vi "ReadWaveDataProcess.vi"(8 "error in (no error)":errorcluster, 11 "ScopeAA in":refnum<class "ScopeAA.lvclass">) -> (0 "error out":errorcluster, 2 "Waveform":waveform(dbl), 3 "ScopeAA out":refnum<class "ScopeAA.lvclass">)   [LabVIEW 2018, in "ScopeAA.lvclass"]
uses:
  ScopeAA.lvclass
  <vilib>/measure/NI_MABase.lvlib
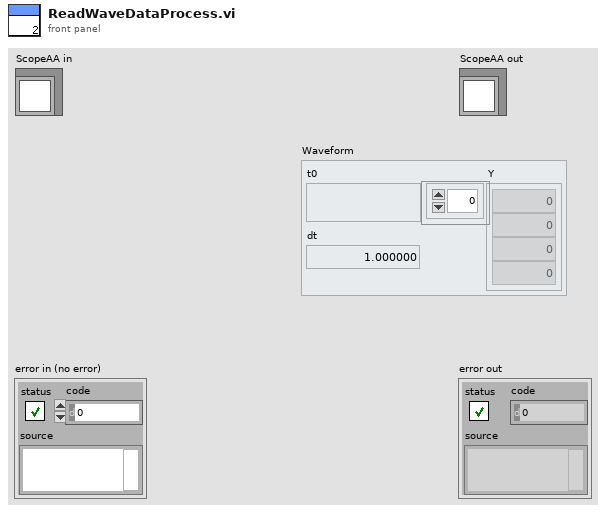
[diagram p1: front panel]
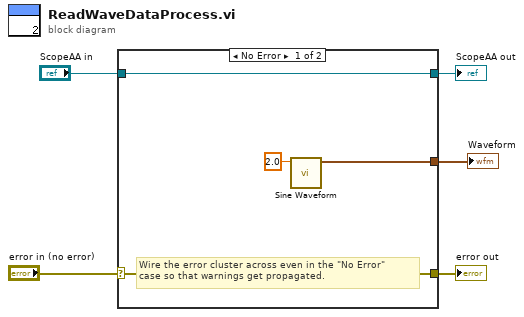
[diagram p0: block diagram]
diagram:
  n1 = case shown="No Error" "error in (no error)" {
    selector: "error in (no error)" -> [w8 w11]
    tunnel: [w8 w11] -> w5
    tunnel: [w9 w10] -> w4
    tunnel: "ScopeAA in" -> [w9 w10]
    tunnel: [w7 _] -> w1
    frame No Error {
      # "Wire the error cluster across even in the \"No Error\"\ncase so that warnings get propagated."
      n2 = call <vilib>:"Sine Waveform.vi"("frequency"=2.0) -> ("signal out"=w7:waveform(dbl))  [unwired: 9 in, 1 out]
    }
    frame Error {
    }
  }
  "error out" <- w5
  "ScopeAA out" <- w4
  "Waveform" <- w1
